vi "Read-from-file-by-value.vi"(8 "error in (no error)":errorcluster, 11 "SettingsFile in":refnum<class "SettingsFile.lvclass">) -> (0 "error out":errorcluster, 2 "Values read":T1, 3 "SettingsFile out":refnum<class "SettingsFile.lvclass">)   [LabVIEW 2013, in "SettingsFile.lvlib" / "SettingsFile.lvclass"]
uses:
  SettingsFile.lvclass
  Values-to-save.ctl
  SettingsFile.lvclass/SettingsFile.ctl
  Errors.ctl
  <vilib>/Utility/xml.llb/Read From XML File(string).vi
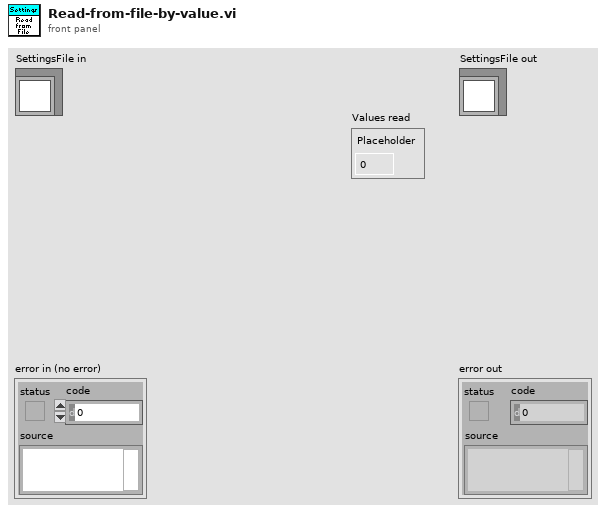
[diagram p1: front panel]
types:
  T1 = typedef "SettingsFile.lvlib/SettingsFile.lvclass/Values-to-save.ctl" = cluster{"Placeholder":dbl}
  T2 = typedef "SettingsFile.lvlib/SettingsFile.lvclass/Errors.ctl" = enum16{"Not implemented", "Command not recognized", "Invalid input", "No connection", "Timeout", "Invalid file type", "No file access"}
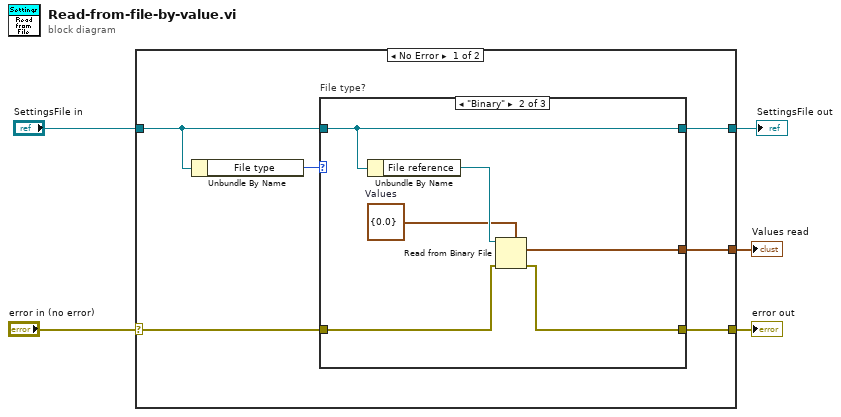
[diagram p0: block diagram]
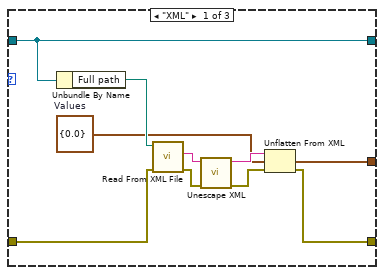
[diagram p2: hidden frame]
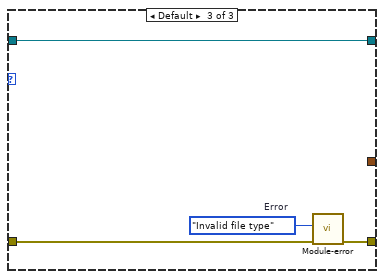
[diagram p3: hidden frame]
diagram:
  n1 = case shown="No Error" "error in (no error)" {
    selector: "error in (no error)" -> [w8 w33]
    tunnel: [w7 w33] -> w4
    tunnel: [w9 w32] -> w2
    tunnel: "SettingsFile in" -> [w10 w32]
    tunnel: [w6 _] -> w1
    frame No Error {
      n2 = Unbundle By Name(w10) -> ("File type"=w11:enum16{"XML", "INI", "Binary"})
      n3 = case "File type?" shown="\"Binary\"" w11 {
        tunnel: w10 -> [w20 w27 w31]
        tunnel: [w20 w27 w31] -> w9
        tunnel: w8 -> [w15 w25 w29]
        tunnel: [w12 w24 w30] -> w7
        tunnel: [w16 w22 _] -> w6
        frame "XML" {
          w17 = T1 {"Placeholder"=0.0}  # Values
          n4 = Unbundle By Name(w20) -> ("Full path"=w21:path)
          n5 = call-poly <vilib>:"Read From XML File.vi"("error in (no error)"=w15, "XML File Path"=w21) -> ("error out"=w14:errorcluster, "XML Elements"=w19:string)  [unwired: 7 in, 1 out]
          n6 = call <vilib>:"Unescape XML.vi"("error in (no error)"=w14, "XML String In"=w19) -> ("error out"=w13:errorcluster, "XML String Out"=w18:string)  [unwired: 8 in]
          n7 = Unflatten From XML(xml string=w18, type=w17, error in (no error)=w13) -> (value=w16:T1, error out=w12:errorcluster)
        }
        frame "Binary" {
          w23 = T1 {"Placeholder"=0.0}  # Values
          n8 = Unbundle By Name(w27) -> ("File reference"=w26:refnum<file>)
          n9 = Read from Binary File(5:w23, 8:w25, 11:w26) -> (0:w24:errorcluster, 2:w22:T1)  [unwired: 3 in, 2 out]
        }
        frame Default {
          w28 = Errors."Invalid file type"  # Error
          n10 = call "Module-error.vi"("error in (no error)"=w29, "Error"=w28) -> ("error out"=w30:errorcluster)  [unwired: 9 in]
        }
      }
    }
    frame Error {
    }
  }
  "error out" <- w4
  "SettingsFile out" <- w2
  "Values read" <- w1
